vi "KundtsTube.vi"() -> ()   [LabVIEW 2014]
panel:
  in  "Amplitude":dbl
  in  "Frequency":dbl
  out "RMS":dbl
  in  "Input":T1
  in  "# of Samples":dbl
  in  "Sampling Rate":dbl
  out "Waveform: Amplitude vs. Time":dynamicdata(graph)
  out "Gain vs. Frequency":cluster{"X":dbl, "Y":dbl}[](graph)
  in  "?":enum32{"Sweep", "Single"}(tab)
  in  "Dwell Time":dbl
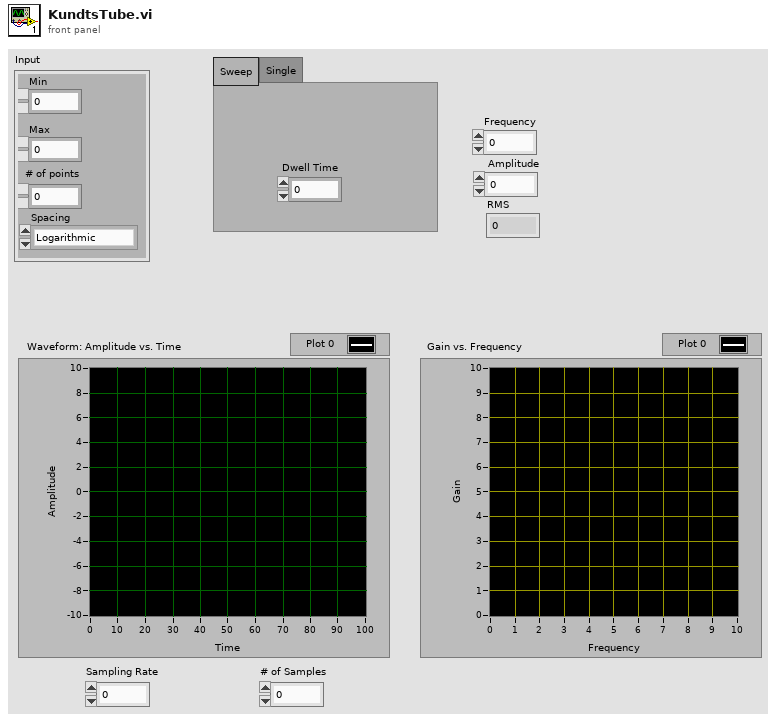
[diagram p1: front panel]
types:
  T1 = cluster{"Min":dbl, "Max":dbl, "# of points":dbl, "Spacing":enum16{"Logarithmic", "Linear"}}
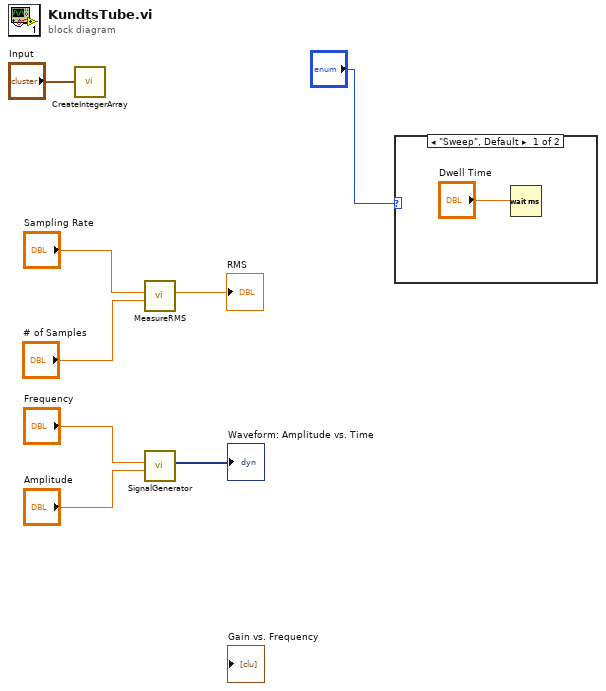
[diagram p0: block diagram]
diagram:
  n1 = call "CreateIntegerArray.vi"("Input"="Input") -> ()  [unwired: 10 in, 1 out]
  n2 = call "MeasureRMS.vi"("# of Samples"="# of Samples", "Sampling Rate"="Sampling Rate") -> ("RMS"=→"RMS":dbl)  [unwired: 8 in, 1 out]
  n3 = call "SignalGenerator.vi"("Amplitude"="Amplitude", "Frequency"="Frequency") -> ("Sine"=→"Waveform: Amplitude vs. Time":dynamicdata)  [unwired: 9 in]
  n4 = case shown="\"Sweep\", Default" "?" {
    frame "Sweep", Default {
      n5 = Wait (ms)(milliseconds to wait="Dwell Time") -> ()  [unwired: 1 out]
    }
    frame "Single" {
    }
  }
